vi "NI6071E_RT_Export Waveform.vi"(4 "Header? (write header:T)":bool=TRUE, 5 "delimiter (Tab)":string="\t", 6 "append to file? (new file:F)":bool, 7 "prompt":string="Choose file to write.", 8 "error in (no error)":errorcluster, 9 "multiple time columns? (single:F)":bool, 10 "Waveforms":waveform(dbl)[](array[waveform]), 11 "file path (dialog if empty)":path) -> (0 "error out":errorcluster, 3 "new file path (Not A Path if cancelled)":path)   [LabVIEW 2009]
doc: "Converts a waveform to a text string and writes the string to a new byte stream file or appends the string to an existing file. You optionally can transpose the data. You can use this polymorphic VI to convert a 1D array of waveforms, a 2D array of waveforms, or a single waveform to a text string. The data type you wire to the <B>Waveform</B> input determines the polymorphic instance to use."
uses:
  <vilib>/Waveform/WDTOps.llb/WDT Get Waveform Time Array DBL.vi
panel:
  out "Array":string[](array[string])
  out "spreadsheet string":string
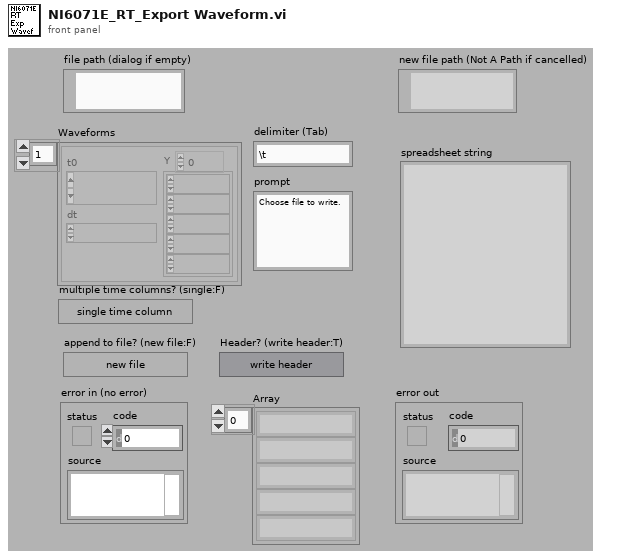
[diagram p1: front panel]
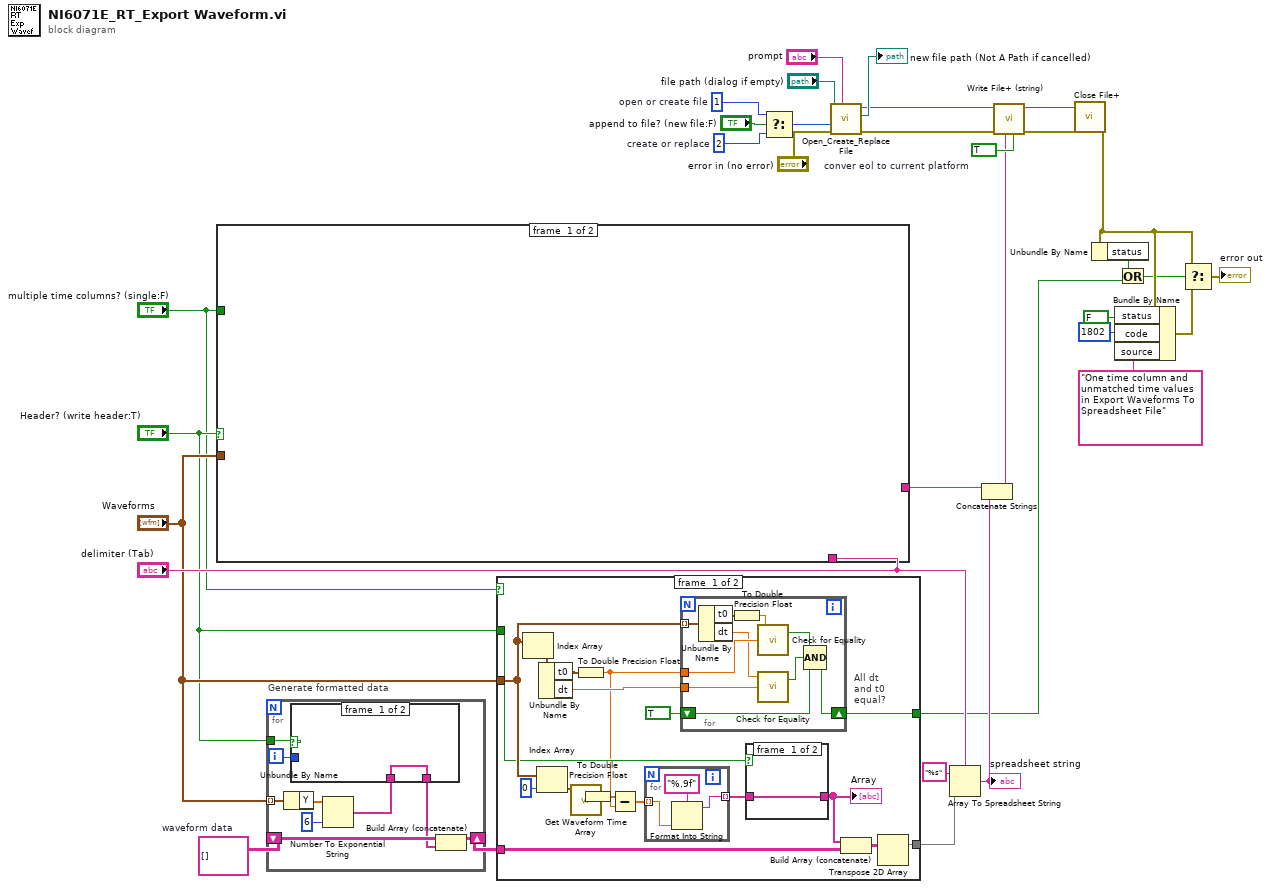
[diagram p0: block diagram]
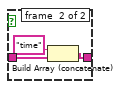
[diagram p2: hidden frame]
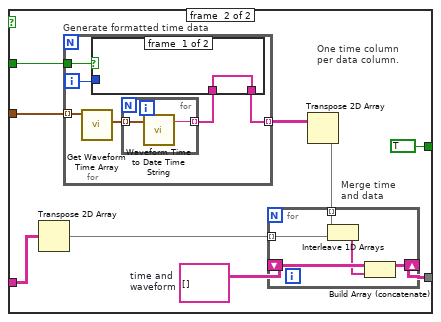
[diagram p3: hidden frame]
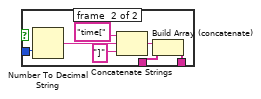
[diagram p4: hidden frame]
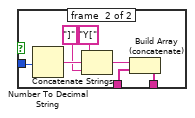
[diagram p5: hidden frame]
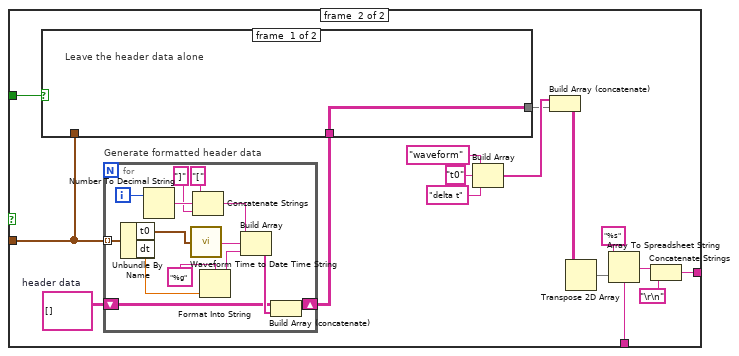
[diagram p6: hidden frame]
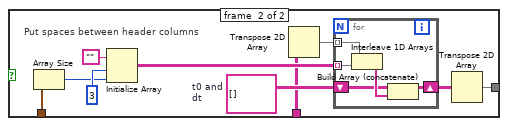
[diagram p7: hidden frame]
diagram:
  w15 = string[][] []  # waveform data
  w25 = i16 2  # create or replace
  w27 = TRUE  # conver eol to current platform
  w32 = i16 1  # open or create file
  n1 = case shown="True" "Header? (write header:T)" {
    tunnel: "delimiter (Tab)" -> [_ w47]
    tunnel: "Waveforms" -> [_ w40]
    tunnel: [_ w41] -> w16
    tunnel: "multiple time columns? (single:F)" -> [_ w38]
    frame #0 {
    }
    frame #1 {
      w44 = string[][] []  # header data
      n2 = for "Generate formatted header data" {
        shift-right: [w68] -> w36
        shift-left: w44 -> [w69]
        tunnel: w40 -> [w71] mode=indexing
        i -> [w74]
        n3 = Unbundle By Name(w71) -> ("t0"=w66:timestamp, "dt"=w77:dbl)
        n4 = Number To Decimal String(number=w74) -> (decimal integer string=w75:string)  [unwired: 1 in]
        n5 = call <vilib>:"Waveform Time to Date Time String.vi"("t0"=w66) -> ("String"=w78:string)
        n6 = Concatenate Strings("[", w75, "]") -> (w76:string)
        n7 = Format Into String(format string="%g" ("Format String"), w77) -> (resulting string=w79:string)  [unwired: 2 in, 1 out]
        n8 = Build Array(w76, w78, w79) -> (w70:string[])
        n9 = Build Array (concatenate)(w69, w70) -> (w68:string[][])
      }
      n10 = case shown="True" w38 {
        tunnel: w40 -> [_ w60]
        tunnel: [w50 w55] -> w37
        tunnel: w36 -> [w50 w54]
        frame #0 {
          # "Leave the header data alone"
        }
        frame #1 {
          w58 = string[][] []  # t0 and dt
          # "Put spaces between header columns"
          n11 = Array Size(array=w60) -> (size(s)=w51:i32)
          n12 = Initialize Array("", 3 ("Dimension Size"), w51) -> (w57:string[][])
          n13 = Transpose 2D Array(2D array=w54) -> (transposed array=w53:string[][])
          n14 = for {
            shift-right: [w62] -> w56
            shift-left: w58 -> [w63]
            tunnel: w57 -> [w65] mode=indexing
            tunnel: w53 -> [w61] mode=indexing
            n15 = Interleave 1D Arrays(w61, w65) -> (w64:string[])
            n16 = Build Array (concatenate)(w63, w64) -> (w62:string[][])
          }
          n17 = Transpose 2D Array(2D array=w56) -> (transposed array=w55:string[][])
        }
      }
      n18 = Build Array("waveform", "t0", "delta t") -> (w39:string[])
      n19 = Build Array (concatenate)(w39, w37) -> (w34:string[][])
      n20 = Transpose 2D Array(2D array=w34) -> (transposed array=w35:string[][])
      n21 = Array To Spreadsheet String(delimiter (Tab)=w47, array=w35, 3:"%s" ("format string")) -> (spreadsheet string=w43:string)
      n22 = Concatenate Strings(w43, "\r\n") -> (w41:string)
    }
  }
  n23 = for "Generate formatted data" {
    tunnel: "Waveforms" -> [w86] mode=indexing
    shift-right: [w83] -> w14
    shift-left: w15 -> [w84]
    tunnel: "Header? (write header:T)" -> [w82]
    i -> [w85]
    n24 = Unbundle By Name(w86) -> ("Y"=w88:dbl[])
    n25 = Number To Exponential String(number=w88, precision (6)=i16 6) -> (E-format string=w81:string[])  [unwired: 2 in]
    n26 = case shown="True" w82 {
      tunnel: w85 -> [_ w93]
      tunnel: w81 -> [w89 w91]
      tunnel: [w89 w90] -> w80
      frame #0 {
      }
      frame #1 {
        n27 = Number To Decimal String(number=w93) -> (decimal integer string=w96:string)  [unwired: 1 in]
        n28 = Concatenate Strings("Y[", w96, "]") -> (w92:string)
        n29 = Build Array (concatenate)(w92, w91) -> (w90:string[])
      }
    }
    n30 = Build Array (concatenate)(w84, w80) -> (w83:string[][])
  }
  n31 = case shown="True" "multiple time columns? (single:F)" {
    tunnel: "Waveforms" -> [w105 w140]
    tunnel: w14 -> [w111 w138]
    tunnel: [w109 w134] -> w13
    tunnel: [w104 TRUE] -> w3
    tunnel: "Header? (write header:T)" -> [w101 w132]
    frame #0 {
      # "One time column - check for equal dt and t0"
      # "All dt\nand t0\nequal?"
      n32 = Index Array(array=w105) -> (element=w108:waveform(dbl))  [unwired: 1 in]
      n33 = Index Array(array=w105, index=0 ("Index")) -> (element=w113:waveform(dbl))
      n34 = Unbundle By Name(w108) -> ("t0"=w103:timestamp, "dt"=w106:dbl)
      n35 = call-poly <vilib>:"Get Waveform Time Array.vi"("waveform in"=w113) -> ("X array"=w97:timestamp[])  [unwired: 9 in, 1 out]
      n36 = To Double Precision Float(number=w103) -> (double precision float=w99:dbl)
      n37 = To Double Precision Float(number=w97) -> (double precision float=w100:dbl[])
      n38 = Subtract(x=w100, y=w99) -> (x-y=w98:dbl[])
      n39 = for {
        tunnel: w98 -> [w131] mode=indexing
        tunnel: [w130] -> w112 mode=indexing
        n40 = Format Into String(format string="%.9f", w131) -> (resulting string=w130:string)  [unwired: 2 in, 1 out]
      }
      n41 = for {
        tunnel: w105 -> [w128] mode=indexing
        shift-right: [w123] -> w104
        shift-left: TRUE -> [w122]
        tunnel: w99 -> [w126]
        tunnel: w106 -> [w124]
        n42 = Unbundle By Name(w128) -> ("t0"=w119:timestamp, "dt"=w125:dbl)
        n43 = To Double Precision Float(number=w119) -> (double precision float=w127:dbl)
        n44 = call <vilib>:"Check for Equality.vi"("n2"=w126, "n1"=w127) -> ("equal?"=w120:bool)  [unwired: 1 in, 1 out]
        n45 = call <vilib>:"Check for Equality.vi"("n2"=w124, "n1"=w125) -> ("equal?"=w121:bool)  [unwired: 1 in, 1 out]
        n46 = Compound Arithmetic op=AND(w120, w121, w122) -> (w123:bool)
      }
      n47 = case shown="True" w101 {
        tunnel: w112 -> [w115 w118]
        tunnel: [w115 w117] -> w102
        frame #0 {
        }
        frame #1 {
          n48 = Build Array (concatenate)("time", w118) -> (w117:string[])
        }
      }
      "Array" <- w102
      n49 = Build Array (concatenate)(w102, w111) -> (w110:string[][])
      n50 = Transpose 2D Array(2D array=w110) -> (transposed array=w109:string[][])
    }
    frame #1 {
      w135 = string[][] []  # time and waveform
      # "One time column\nper data column."
      n51 = Transpose 2D Array(2D array=w138) -> (transposed array=w137:string[][])
      n52 = for "Generate formatted time data" {
        tunnel: [w147] -> w139 mode=indexing
        tunnel: w140 -> [w151] mode=indexing
        tunnel: w132 -> [w149]
        i -> [w150]
        n53 = call-poly <vilib>:"Get Waveform Time Array.vi"("waveform in"=w151) -> ("X array"=w146:timestamp[])  [unwired: 9 in, 1 out]
        n54 = for {
          tunnel: w146 -> [w160] mode=indexing
          tunnel: [w161] -> w148 mode=indexing
          n55 = call <vilib>:"Waveform Time to Date Time String.vi"("t0"=w160) -> ("String"=w161:string)
        }
        n56 = case shown="False" w149 {
          tunnel: w150 -> [_ w156]
          tunnel: w148 -> [w152 w154]
          tunnel: [w152 w153] -> w147
          frame #0 {
          }
          frame #1 {
            n57 = Number To Decimal String(number=w156) -> (decimal integer string=w159:string)  [unwired: 1 in]
            n58 = Concatenate Strings("time[", w159, "]") -> (w155:string)
            n59 = Build Array (concatenate)(w155, w154) -> (w153:string[])
          }
        }
      }
      n60 = Transpose 2D Array(2D array=w139) -> (transposed array=w136:string[][])
      n61 = for "Merge time\nand data" {
        tunnel: w137 -> [w144] mode=indexing
        tunnel: w136 -> [w143] mode=indexing
        shift-right: [w142] -> w134
        shift-left: w135 -> [w145]
        n62 = Interleave 1D Arrays(w143, w144) -> (w141:string[])
        n63 = Build Array (concatenate)(w145, w141) -> (w142:string[][])
      }
    }
  }
  n64 = Select ("function")(t=w32, s="append to file? (new file:F)", f=w25) -> (s? t:f=w30:i16)
  n65 = call <vilib>:"Open_Create_Replace File.vi"("prompt"="prompt", "error in (no error)"="error in (no error)", "function (open:0)"=w30, "file path"="file path (dialog if empty)") -> ("error out"=w20:errorcluster, "new file path"=→"new file path (Not A Path if cancelled)":path, "refnum"=w19:refnum<file>)  [unwired: 4 in, 1 out]
  n66 = Array To Spreadsheet String(delimiter (Tab)="delimiter (Tab)", array=w13, 3:"%s" ("format (%.3f)")) -> (spreadsheet string=w18:string)
  "spreadsheet string" <- w18
  n67 = Concatenate Strings(w16, w18) -> (w17:string)
  n68 = call <vilib>:"Write File+ (string).vi"("convert eol? (no:F)"=w27, "string"=w17, "error in (no error)"=w20, "refnum"=w19) -> ("error out"=w31:errorcluster, "dup refnum"=w28:refnum<file>)  [unwired: 3 in, 1 out]
  n69 = call <vilib>:"Close File+.vi"("error in (no error)"=w31, "refnum"=w28) -> ("error out"=w10:errorcluster)  [unwired: 3 in, 2 out]
  n70 = Unbundle By Name(w10) -> ("status"=w9:bool)
  n71 = Bundle By Name(cluster=w10, "status"=FALSE, "code"=1802, "source"="One time column and unmatched time values in Export Waveforms To Spreadsheet File") -> (w11:errorcluster)
  n72 = Or(x=w9, y=w3) -> (x .or. y?=w8:bool)
  n73 = Select(t=w10, s=w8, f=w11) -> (s? t:f=→"error out":errorcluster)
